vi "Download File with Callback.vi"(8 "error in (no error)":errorcluster, 9 "Connection Name":string, 10 "Local File Path":path, 11 "Remote File Path":string) -> (0 "error out":errorcluster, 3 "Return String":string)   [LabVIEW 2015, in "LabSFTP.lvlib"]
doc: "<License>This software is distributed under the BSD 3-Clause License. For the full license please see license.txt or visit www.labvolution.com/license</License>"
uses:
  LabSFTP.lvlib
  FGV State..enum.ctl
  C:/Working Folder/ssh.git/LabSSH Library/References/LabSFTP.dll
  References/LabSFTP.dll
  DownloadStatus..Callback.vi
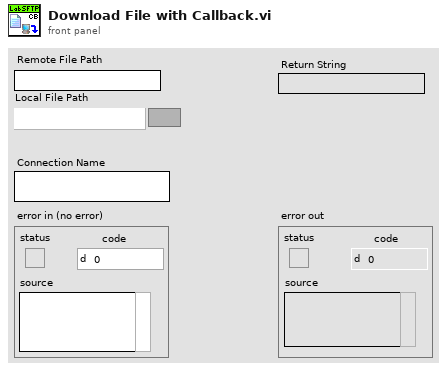
[diagram p1: front panel]
types:
  T1 = typedef "LabSFTP.lvlib/FGV State..enum.ctl" = enum16{"GET", "SET"}
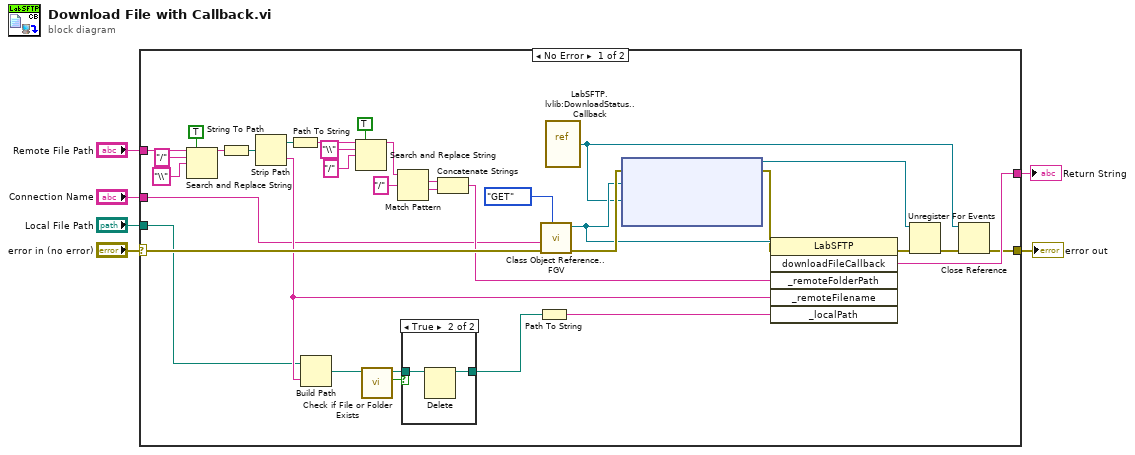
[diagram p0: block diagram]
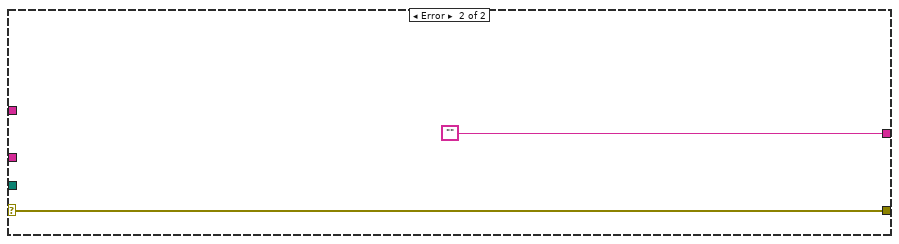
[diagram p3: hidden frame]
diagram:
  n1 = case shown="No Error" "error in (no error)" {
    selector: "error in (no error)" -> [w41 w46]
    tunnel: [w8 w46] -> w5
    tunnel: [w38 ""] -> w4
    tunnel: "Local File Path" -> [w16 _]
    tunnel: "Remote File Path" -> [w22 _]
    tunnel: "Connection Name" -> [w14 _]
    frame No Error {
      n2 = Search and Replace String(replace all?=TRUE ("replace all? (F)"), input string=w22, search string="/", replace string="\\" ("replace string (\"\")")) -> (result string=w26:string)  [unwired: 4 in, 3 out]
      n3 = String To Path(string=w26) -> (path=w27:path)
      n4 = Strip Path(path=w27) -> (stripped path=w28:path, name=w17:string)
      n5 = Path To String(path=w28) -> (string=w32:string)
      n6 = Build Path(base path=w16, name or relative path=w17) -> (appended path=w15:path)
      n7 = Search and Replace String(replace all?=TRUE ("replace all? (F)"), input string=w32, search string="\\", replace string="/" ("replace string (\"\")")) -> (result string=w34:string)  [unwired: 4 in, 3 out]
      n8 = call <vilib>:"Check if File or Folder Exists.vi"("path"=w15) -> ("file or folder exists?"=w20:bool, "dup path"=w19:path)  [unwired: 8 in, 1 out]
      n9 = Match Pattern(string=w34, regular expression="/") -> (match substring=w35:string, after substring=w36:string)  [unwired: 1 in, 2 out]
      n10 = case shown="True" w20 {
        tunnel: w19 -> [w42 w44]
        tunnel: [w42 w43] -> w18
        frame False {
        }
        frame True {
          n11 = Delete(path (use dialog)=w44) -> (deleted path=w43:path)  [unwired: 4 in, 2 out]
        }
      }
      n12 = Concatenate Strings(w35, w36) -> (w21:string)
      n13 = Path To String(path=w18) -> (string=w37:string)
      n14 = call "Class Object Reference..FGV.vi"("FGV State"=FGV_State..enum."GET", "error in (no error)"=w41, "Connection Name"=w14) -> ("error out"=w13:errorcluster, "LabSFTP ref out"=w12:refnum<k24>)  [unwired: 7 in]
      n15 = vi-ref "LabSFTP.lvlib:DownloadStatus..Callback.vi"() -> (w7:refnum<vi>)
      n16 = node(w13, w12, w7) -> (w9:refnum<k27>, w11:errorcluster)  [unwired: 2 in]
      n17 = invoke class="LabSFTP" method="downloadFileCallback"(reference=w12, error in=w11, "_remoteFolderPath"=w21, "_remoteFilename"=w17, "_localPath"=w37) -> (error out=w39:errorcluster, "downloadFileCallback"=w38:string)  [unwired: 1 in, 4 out]
      n18 = Unregister For Events(event registration refnum=w9, error in=w39) -> (error out=w10:errorcluster)
      n19 = Close Reference(reference=w7, error in (no error)=w10) -> (error out=w8:errorcluster)
    }
    frame Error {
    }
  }
  "error out" <- w5
  "Return String" <- w4
